vi "CrossbowWinch.vi"(10 "Up":bool, 11 "Down":bool) -> (2 "Output 2":dbl)   [LabVIEW 2015]
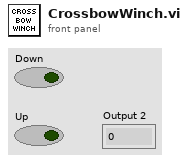
[diagram p1: front panel]
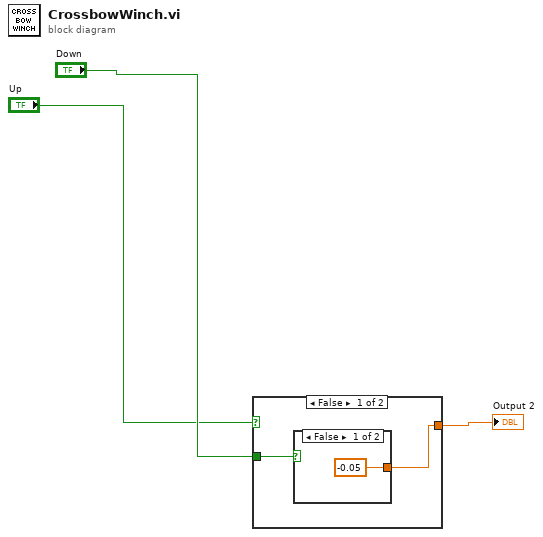
[diagram p0: block diagram]
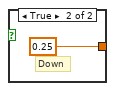
[diagram p2: hidden frame]
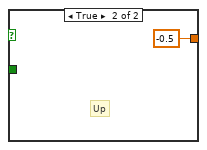
[diagram p3: hidden frame]
diagram:
  n1 = case shown="False" "Up" {
    tunnel: [w5 -0.5 ("Output")] -> w3
    tunnel: "Down" -> [w4 _]
    frame False {
      n2 = case shown="False" w4 {
        tunnel: [-0.05 ("Output") 0.25 ("Output")] -> w5
        frame False {
        }
        frame True {
          # "Down"
        }
      }
    }
    frame True {
      # "Up"
    }
  }
  "Output 2" <- w3
